vi "UA_Initial_Server.vi"(8 "error in (no error)":errorcluster caption="error in", 11 "Server config infor":T1) -> (0 "error out":errorcluster, 3 "OPC UA server refnum out":refnum<k21>, 5 "server endpoint URL":string)   [LabVIEW 2013, in "OPCUA XML.lvlib"]
uses:
  OPCUA XML.lvlib
  UA_Server config info.ctl
  UA_OP Action.ctl
  <vilib>/OPCUA/NI OPC UA Server.lvlib
  <vilib>/OPCUA/server/Read Int32.vi
  <vilib>/OPCUA/server/Write Int32.vi
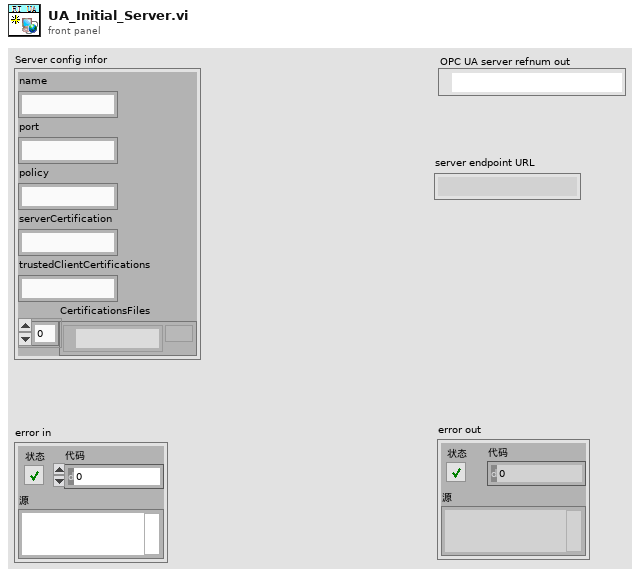
[diagram p1: front panel]
types:
  T1 = typedef "OPCUA XML.lvlib/UA_Server config info.ctl" = cluster{"name":string, "port":string, "policy":string, "serverCertification":string, "trustedClientCertifications":string, "CertificationsFiles":path[]}
  T2 = typedef "OPCUA XML.lvlib/UA_OP Action.ctl" = enum16{"Initial", "Add node", "Get node", "Get length", "View node"}
  T3 = typedef "supported security policies.ctl" = cluster{"None":bool, "Sign with Basic128Rsa125":bool, "Sign and Encrypt with Basic128Rsa125":bool, "Sign with Basic256":bool, "Sign and Encrypt with Basic256":bool}
  T4 = cluster{"name":string, "data type":u16, "access level":u16, "description":string}
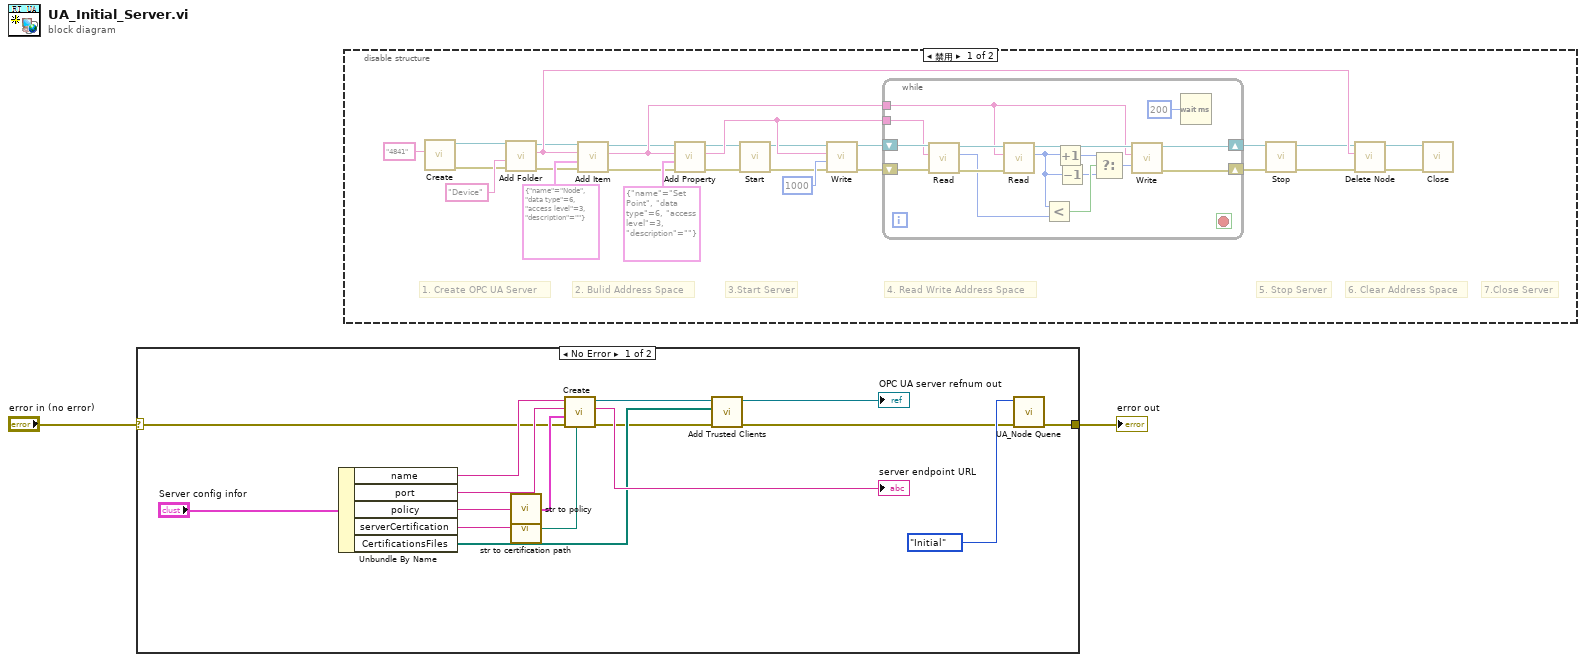
[diagram p0: block diagram]
diagram:
  n1 = case shown="No Error" "error in (no error)" {
    selector: "error in (no error)" -> [w11 w19]
    tunnel: [w3 w19] -> w1
    frame No Error {
      n2 = Unbundle By Name("Server config infor") -> ("name"=w17:string, "port"=w16:string, "policy"=w13:string, "serverCertification"=w15:string, "CertificationsFiles"=w8:path[])
      n3 = call "str to policy.vi"("String"=w13) -> ("supported security policies (None)"=w12:T3)  [unwired: 6 in]
      n4 = call "str to certification path.vi"("node text"=w15) -> ("File Path Control"=w14:path)  [unwired: 4 in]
      n5 = call <vilib>:"Create.vi"("server certificate file"=w14, "error in (no error)"=w11, "supported security policies (None)"=w12, "TCP port (49580)"=w16, "OPC UA server name"=w17) -> ("error out"=w7:errorcluster, "server endpoint URL"=→"server endpoint URL":string, "OPC UA server refnum out"=w9:refnum<k21>)  [unwired: 4 in]
      n6 = call <vilib>:"Add Trusted Clients.vi"("error in (no error)"=w7, "trusted client certificates"=w8, "OPC UA server refnum in"=w9) -> ("error out"=w4:errorcluster, "OPC UA server refnum out"=→"OPC UA server refnum out":refnum<k21>)  [unwired: 7 in]
      n7 = call "UA_Node Quene.vi"("error in (no error)"=w4, "OP Action"=UA_OP_Action."Initial") -> ("error out"=w3:errorcluster)  [unwired: 7 in, 2 out]
    }
    frame Error {
    }
  }
  "error out" <- w1
  n8 = disable-structure shown="禁用" {
    frame Disabled {
      # "7.Close Server"
      # "6. Clear Address Space"
      # "5. Stop Server"
      # "4. Read Write Address Space"
      # "3.Start Server"
      # "2. Bulid Address Space"
      # "1. Create OPC UA Server"
      n9 = call <vilib>:"Create.vi"("TCP port (49580)"="4841" ("TCP port (4840)")) -> ("error out"=w21:errorcluster, "OPC UA server refnum out"=w20:refnum<k21>)  [unwired: 8 in, 1 out]
      n10 = call <vilib>:"Add Folder.vi"("error in (no error)"=w21, "folder name"="Device", "OPC UA server refnum in"=w20) -> ("error out"=w24:errorcluster, "folder path"=w42:string, "OPC UA server refnum out"=w23:refnum<k21>)  [unwired: 5 in]
      n11 = call <vilib>:"Add Item.vi"("error in (no error)"=w24, "item"=T4 {"name"="Node", "data type"=6, "access level"=3, "description"=""}, "parent folder path"=w42, "OPC UA server refnum in"=w23) -> ("error out"=w35:errorcluster, "item path"=w37:string, "OPC UA server refnum out"=w25:refnum<k21>)  [unwired: 4 in]
      n12 = call <vilib>:"Add Property.vi"("error in (no error)"=w35, "property"=T4 {"name"="Set Point", "data type"=6, "access level"=3, "description"=""} ("item"), "item path"=w37, "OPC UA server refnum in"=w25) -> ("error out"=w36:errorcluster, "property path"=w44:string, "OPC UA server refnum out"=w34:refnum<k21>)  [unwired: 4 in]
      n13 = call <vilib>:"Start.vi"("error in (no error)"=w36, "OPC UA server refnum in"=w34) -> ("error out"=w40:errorcluster, "OPC UA server refnum out"=w26:refnum<k21>)  [unwired: 8 in]
      n14 = call-poly <vilib>:"Write.vi"("error in (no error)"=w40, "value"=1000, "node path"=w44, "OPC UA server refnum in"=w26) -> ("error out"=w41:errorcluster, "OPC UA server refnum out"=w39:refnum<k21>)  [unwired: 6 in]
      n15 = while {
        tunnel: w37 -> [w52]
        shift-right: [w58] -> w29
        shift-left: w39 -> [w57]
        shift-right: [w56] -> w31
        shift-left: w41 -> [w60]
        tunnel: w44 -> [w55]
        stop <- w62 stop-if-true
        n16 = call-poly <vilib>:"Read.vi"("error in (no error)"=w60, "node path"=w55, "OPC UA server refnum in"=w57) -> ("error out"=w53:errorcluster, "value"=w51:i32, "OPC UA server refnum out"=w61:refnum<k21>)  [unwired: 4 in, 2 out]
        n17 = call-poly <vilib>:"Read.vi"("error in (no error)"=w53, "node path"=w52, "OPC UA server refnum in"=w61) -> ("value"=w47:i32, "OPC UA server refnum out"=w54:refnum<k21>)  [unwired: 4 in, 3 out]
        n18 = Less?(x=w47, y=w51) -> (x < y?=w50:bool)
        n19 = Increment(x=w47) -> (x+1=w49:i32)
        n20 = Decrement(x=w47) -> (x-1=w48:i32)
        n21 = Select(t=w49, s=w50, f=w48) -> (s? t:f=w46:i32)
        n22 = call-poly <vilib>:"Write.vi"("value"=w46, "node path"=w52, "OPC UA server refnum in"=w54) -> ("error out"=w56:errorcluster, "OPC UA server refnum out"=w58:refnum<k21>)  [unwired: 7 in]
        n23 = Wait (ms)(milliseconds to wait=u32 200) -> ()  [unwired: 1 out]
      }
      n24 = call <vilib>:"Stop.vi"("error in (no error)"=w31, "OPC UA server refnum in"=w29) -> ("error out"=w32:errorcluster, "OPC UA server refnum out"=w30:refnum<k21>)  [unwired: 8 in]
      n25 = call <vilib>:"Delete Node.vi"("error in (no error)"=w32, "node path"=w42, "OPC UA server refnum in"=w30) -> ("error out"=w28:errorcluster, "OPC UA server refnum out"=w27:refnum<k21>)  [unwired: 7 in]
      n26 = call <vilib>:"Close.vi"("error in (no error)"=w28, "OPC UA server refnum in"=w27) -> ()  [unwired: 9 in, 1 out]
    }
    frame Enabled {
    }
  }
